vi "Search_SN_MAC.vi"(11 "MAC&SN":string) -> (2 "MAC":string, 3 "SN":string)   [LabVIEW 2012]
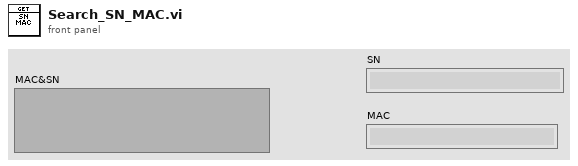
[diagram p1: front panel]
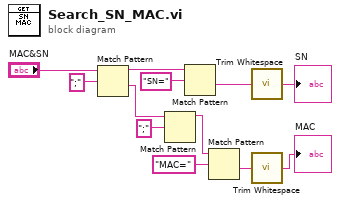
[diagram p0: block diagram]
diagram:
  n1 = Match Pattern(string="MAC&SN", regular expression=";") -> (before substring=w8:string, after substring=w11:string)  [unwired: 1 in, 2 out]
  n2 = Match Pattern(string=w11, regular expression=";") -> (before substring=w5:string)  [unwired: 1 in, 3 out]
  n3 = Match Pattern(string=w8, regular expression="SN=") -> (after substring=w4:string)  [unwired: 1 in, 3 out]
  n4 = Match Pattern(string=w5, regular expression="MAC=") -> (after substring=w2:string)  [unwired: 1 in, 3 out]
  n5 = call <vilib>:"Trim Whitespace.vi"("string"=w4) -> ("trimmed string"=→"SN":string)  [unwired: 1 in]
  n6 = call <vilib>:"Trim Whitespace.vi"("string"=w2) -> ("trimmed string"=→"MAC":string)  [unwired: 1 in]
